vi "FABR-Update Analysis.vi"(0 "Analysis in":T2, 7 "update":T1[](array[typedef]), 11 "error in (no error)":errorcluster) -> (4 "Analysis out":T2, 8 "finished":bool, 15 "error out":errorcluster)   [LabVIEW 2020]
uses:
  Typedefs/FABR-Analysis State.ctl
  Typedefs/FABR-Stimulus Condition.ctl
panel:
  # "Freq X Level X Time"
  # "Freq X Level X Time"
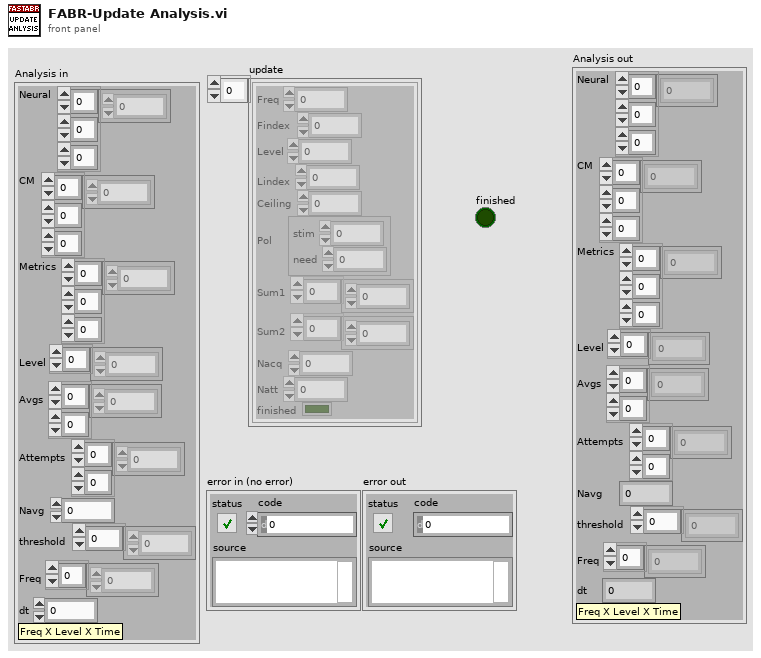
[diagram p1: front panel]
types:
  T1 = typedef "FABR-Stimulus Condition.ctl" = cluster{"Freq":dbl, "Findex":i32, "Level":dbl, "Lindex":i32, "Ceiling":dbl, "Pol":cluster{"stim":i32, "need":i32}, "Sum1":dbl[], "Sum2":dbl[], "Nacq":i32, "Natt":i32, "finished":bool}
  T2 = typedef "FABR-Analysis State.ctl" = cluster{"Neural":dbl[][][], "CM":dbl[][][], "Metrics":dbl[][][], "Level":dbl[], "Avgs":i32[][], "Attempts":i32[][], "Navg":i32, "threshold":dbl[], "Freq":dbl[], "dt":dbl}
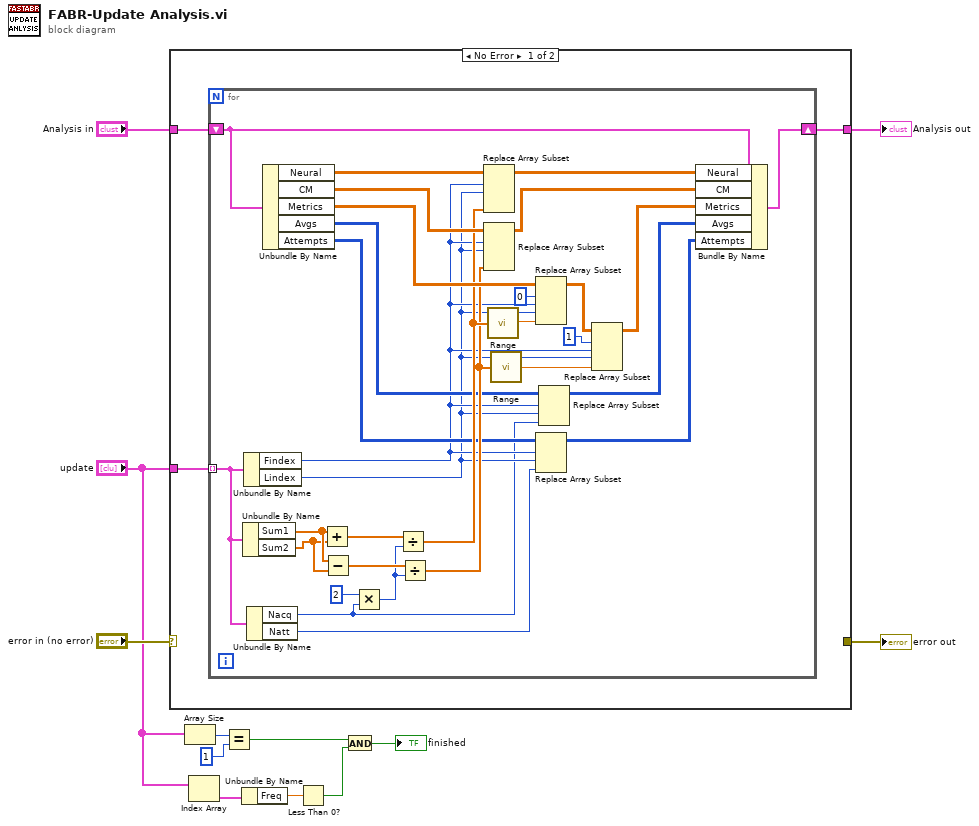
[diagram p0: block diagram]
diagram:
  n1 = case shown="No Error" "error in (no error)" {
    selector: "error in (no error)" -> [_ w47]
    tunnel: "update" -> [w15 _]
    tunnel: "Analysis in" -> [w14 w46]
    tunnel: [w13 w46] -> w11
    tunnel: [_ w47] -> w9
    frame No Error {
      n2 = for {
        tunnel: w15 -> [w40] mode=indexing
        shift-right: [w35] -> w13
        shift-left: w14 -> [w38]
        n3 = Unbundle By Name(w40) -> ("Sum1"=w44:dbl[], "Sum2"=w43:dbl[])
        n4 = Unbundle By Name(w40) -> ("Findex"=w22:i32, "Lindex"=w21:i32)
        n5 = Unbundle By Name(w40) -> ("Nacq"=w17:i32, "Natt"=w20:i32)
        n6 = Unbundle By Name(w38) -> ("Neural"=w41:dbl[][][], "CM"=w39:dbl[][][], "Metrics"=w34:dbl[][][], "Avgs"=w25:i32[][], "Attempts"=w23:i32[][])
        n7 = Add(x=w44, y=w43) -> (x+y=w45:dbl[])
        n8 = Subtract(x=w44, y=w43) -> (x-y=w42:dbl[])
        n9 = Multiply(x=2, y=w17) -> (x*y=w18:i32)
        n10 = Divide(x=w45, y=w18) -> (x/y=w33:dbl[])
        n11 = Divide(x=w42, y=w18) -> (x/y=w30:dbl[])
        n12 = Replace Array Subset(array=w41, new element=w33, index (dim 0)=w22, index (dim 1)=w21) -> (w37:dbl[][][])  [unwired: 1 in]
        n13 = Replace Array Subset(array=w39, new element=w30, index (dim 0)=w22, index (dim 1)=w21) -> (w36:dbl[][][])  [unwired: 1 in]
        n14 = call "Range.vi"("Array"=w33) -> ("Range"=w31:dbl)
        n15 = call "Range.vi"("Array"=w30) -> ("Range"=w27:dbl)
        n16 = Replace Array Subset(array=w34, new element=w31, index (dim 0)=0 ("disabled index (page)"), index (dim 1)=w22, index (dim 2)=w21) -> (w29:dbl[][][])
        n17 = Replace Array Subset(array=w23, new element=w20, index (row)=w22, index (col)=w21) -> (w19:i32[][])
        n18 = Replace Array Subset(array=w25, new element=w17, index (row)=w22, index (col)=w21) -> (w24:i32[][])
        n19 = Replace Array Subset(array=w29, new element=w27, index (dim 0)=1 ("disabled index (page)"), index (dim 1)=w22, index (dim 2)=w21) -> (w28:dbl[][][])
        n20 = Bundle By Name(cluster=w38, "Neural"=w37, "CM"=w36, "Metrics"=w28, "Avgs"=w24, "Attempts"=w19) -> (w35:T2)
      }
    }
    frame Error {
    }
  }
  "Analysis out" <- w11
  "error out" <- w9
  n21 = Array Size(array="update") -> (size(s)=w8:i32)
  n22 = Index Array(array="update") -> (element=w5:T1)  [unwired: 1 in]
  n23 = Equal?(x=w8, y=1) -> (x = y?=w2:bool)
  n24 = Unbundle By Name(w5) -> ("Freq"=w4:dbl)
  n25 = Less Than 0?(x=w4) -> (x < 0?=w3:bool)
  n26 = And(x=w2, y=w3) -> (x .and. y?=→"finished":bool)
